vi "main-launcher.vi"(8 "error in (no error)":errorcluster) -> (0 "error out":errorcluster)   [LabVIEW 2021]
uses:
  Libraries/Interface-Module/Interface-Module.lvlib
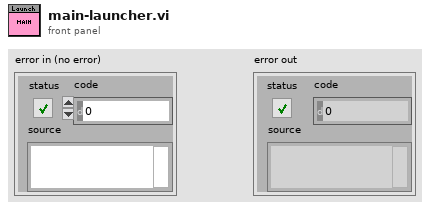
[diagram p1: front panel]
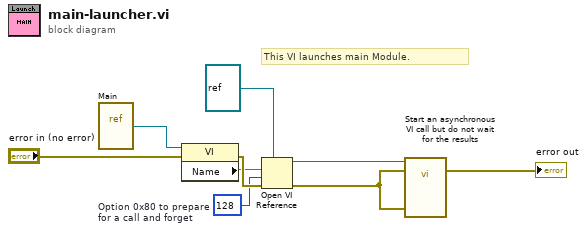
[diagram p0: block diagram]
diagram:
  w7 = 128  # Option 0x80 to prepare for a call and forget
  # "This VI launches main Module."
  n1 = vi-ref "Main.vi"() -> (w2:refnum<vi>)
  n2 = property class="VI"(reference=w2, error in="error in (no error)") -> (error out=w8:errorcluster, "Name"=w5:string)  [unwired: 1 out]
  n3 = Open VI Reference(type specifier VI Refnum (for type only)=refnum<vi> refnum, vi path=w5, options=w7, error in (no error)=w8) -> (vi reference=w6:refnum<vi>, error out=w9:errorcluster)  [unwired: 2 in]
  n4 = call-by-ref "Start an asynchronous\nVI call but do not wait\nfor the results"(reference=w6, error in=w9, "error in"=w9) -> (error out=→"error out":errorcluster)  [unwired: 10 in, 2 out]
